vi "niFPGA_U16 Divide (U8).vi"(2 "D [U16.n]":u16, 3 "N [U16.n]":u16) -> (1 "N/D [U8.0]":u8 format="%.0x")   [LabVIEW 2017]
uses:
  <vilib>/Platform/TimedLoop/XDataNode/timing_clust.ctl
  <vilib>/Platform/TimedLoop/XDataNode/nitl_modes.ctl
  <vilib>/Platform/TimedLoop/XDataNode/wakeup.ctl
  <vilib>/Platform/TimedLoop/XDataNode/XDataNode.xnode
  <vilib>/Platform/TimedLoop/XDataNode/XDNodeRunTimeDep.lvlib
panel:
  # "N <= D"
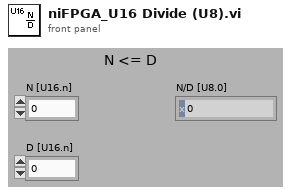
[diagram p1: front panel]
types:
  T1 = typedef "XDNodeRunTimeDep.lvlib/timing_clust.ctl" = cluster{"Expected End [f-1]":u64, "Actual End [f-1]":u64, "Finished Late? [f-1]":bool, "Expected End [i-1]":u64, "Actual End [i-1]":u64, "Finished Late? [i-1]":bool, "Expected Start [i]":u64, "Actual Start [i]":u64, "Expected Start [f]":u64, "Actual Start [f]":u64, "Source Name":string, "Structure Name":string, "Period":i64, "Deadline":i64, "Offset":i64, "Start":i64, "Priority":i32, "Timeout":i32, "Mode":T2, "Wakeup Reason":T3, "Error":errorcluster, "Source Type":string, "Secondary Source Type":string, "Global End Time":u64, "Global Start Time":u64, "Frame Duration":u64, "Iteration Duration":u64, "Assigned CPU":i32, "I/O Scan Engine Mode":u32}
  T2 = typedef "XDNodeRunTimeDep.lvlib/nitl_modes.ctl" = enum32{"No Change", "Process missed periods, maintain original phase", "Discard missed periods, maintain original phase", "Process missed periods, ignore original phase", "Discard missed periods, ignore original phase"}
  T3 = typedef "XDNodeRunTimeDep.lvlib/wakeup.ctl" = enum32{"Normal", "Aborted", "Asynchronous wakeup", "Timing source error", "Timed loop error", "Timeout"}
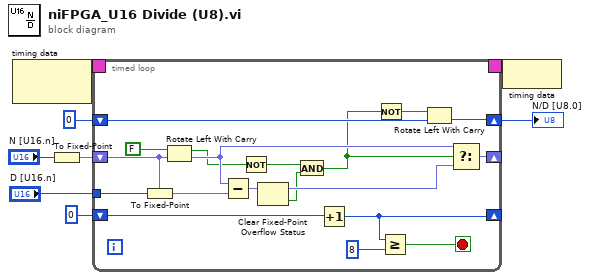
[diagram p0: block diagram]
diagram:
  n1 = node-c288() -> (w8:T1)  [unwired: 1 out]
  n2 = To Fixed-Point(number="N [U16.n]") -> (fixed-point=w2:fxp<+,16,16>)  [unwired: 1 out]
  n3 = timed-loop {
    shift-right: [w23] -> _
    shift-left: w2 -> [w9]
    tunnel: "D [U16.n]" -> [w10]
    shift-right: [w26] -> _
    shift-left: u8 0 -> [w27]
    timing: w8 -> [_]
    timing-out: [_] -> w7
    shift-right: [w22] -> w6
    shift-left: u8 0 -> [w19]
    stop <- w24 stop-if-true
    n4 = To Fixed-Point(fixed-point type=w9, number=w10) -> (fixed-point=w11:fxp<+,16,16>)
    n5 = Rotate Left With Carry(2:w9, 3:FALSE ("carry")) -> (0:w21:fxp<+,16,16>, 1:w17:bool)
    n6 = Subtract(x=w21, y=w11) -> (x-y=w14:fxp<+,16,16>)
    n7 = Not(x=w17) -> (.not. x?=w16:bool)
    n8 = Clear Fixed-Point Overflow Status(3:w14) -> (0:w12:bool, 1:w13:fxp<+,16,16>)
    n9 = And(x=w16, y=w12) -> (x .and. y?=w15:bool)
    n10 = Increment(x=w27) -> (x+1=w26:u8)
    n11 = Not(x=w15) -> (.not. x?=w20:bool)
    n12 = Greater Or Equal?(x=w26, y=u8 8) -> (x >= y?=w24:bool)
    n13 = Rotate Left With Carry(2:w19, 3:w20) -> (0:w22:u8)  [unwired: 1 out]
    n14 = Select(t=w21, s=w15, f=w13) -> (s? t:f=w23:fxp<+,16,16>)
  }
  "N/D [U8.0]" <- w6
  n15 = node-c288(w7) -> ()
